vi "ReadConfigCuster.vi"(2 "error in (no error)":errorcluster, 3 "Ctrl Reference":refnum<vi>, 4 "ConfigFile (input)":T1) -> (0 "error out":errorcluster, 1 "ConfigFile (output)":T1)   [LabVIEW 2009]
uses:
  <vilib>/Utility/config.llb/Config Data RefNum.ctl
  Read Key (Double).vi
  Read Key (Boolean).vi
  Read Key (Path).vi
  Read Key (String).vi
  <vilib>/Utility/config.llb/NI_LVConfig.lvlib
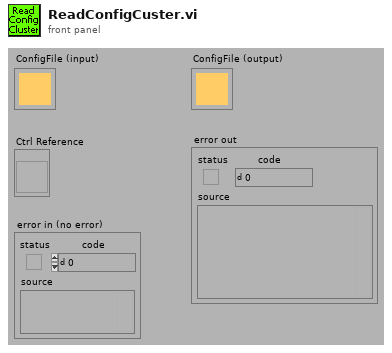
[diagram p1: front panel]
types:
  T1 = typedef "NI_LVConfig.lvlib/Config Data RefNum.ctl" = refnum<k1>
  T2 = typedef "Config Data RefNum" = refnum<k1>
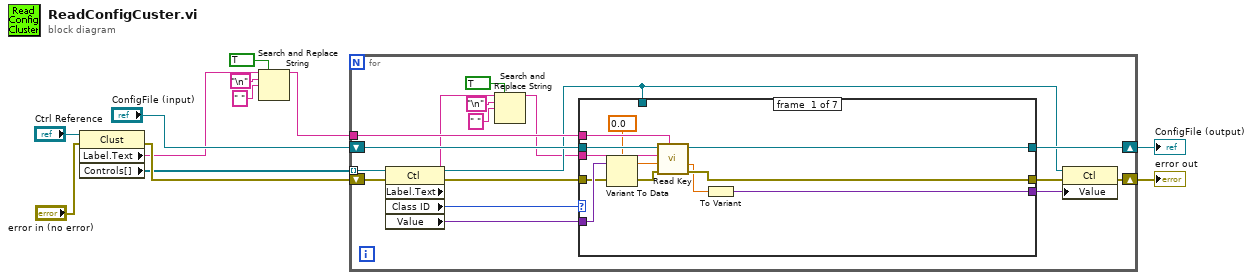
[diagram p0: block diagram]
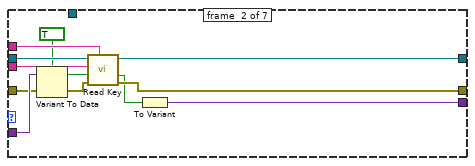
[diagram p2: hidden frame]
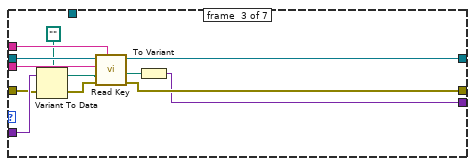
[diagram p3: hidden frame]
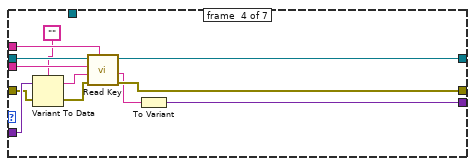
[diagram p4: hidden frame]
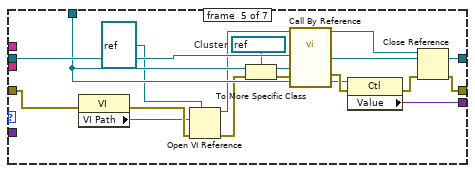
[diagram p5: hidden frame]
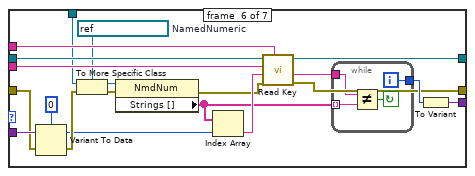
[diagram p6: hidden frame]
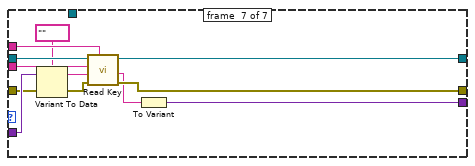
[diagram p7: hidden frame]
diagram:
  n1 = property on="Property Node" class="Clust"(reference="Ctrl Reference", error in="error in (no error)") -> (error out=w8:errorcluster, "Label.Text"=w2:string, "Controls[]"=w6:refnum<vi>[])  [unwired: 1 out]
  n2 = Search and Replace String(replace all?=TRUE ("replace all? (F)"), input string=w2, search string="\n", replace string=" ") -> (result string=w1:string)  [unwired: 4 in, 3 out]
  n3 = for {
    tunnel: w6 -> [w27] mode=indexing
    tunnel: w1 -> [w28]
    shift-right: [w23] -> w9
    shift-left: "ConfigFile (input)" -> [w24]
    shift-right: [w19] -> w12
    shift-left: w8 -> [w22]
    n4 = property on="Property Node" class="Ctl"(reference=w27, error in=w22) -> (reference out=w18:refnum<vi>, error out=w29:errorcluster, "Label.Text"=w14:string, "Class ID"=w26:u32, "Value"=w25:variant)
    n5 = Search and Replace String(replace all?=TRUE ("replace all? (F)"), input string=w14, search string="\n", replace string=" ") -> (result string=w13:string)  [unwired: 4 in, 3 out]
    n6 = case shown="27" w26 {
      tunnel: w24 -> [w41 w53 w65 w77 w94 w112 w130]
      tunnel: w29 -> [w36 w49 w61 w73 w90 w113 w126]
      tunnel: w28 -> [w40 w52 w64 w76 _ w109 w129]
      tunnel: w13 -> [w39 w51 w63 w75 _ w111 w128]
      tunnel: w25 -> [w38 w50 w62 w74 _ w114 w127]
      tunnel: [w34 w47 w59 w71 w91 w105 w124] -> w23
      tunnel: [w33 w46 w58 w70 w80 w98 w123] -> w20
      tunnel: [w31 w43 w54 w67 w89 w102 w120] -> w21
      tunnel: w18 -> [_ _ _ _ w87 w106 _]
      frame #0 {
        n7 = Variant To Data(error in=w36, Variant=w38, type=0.0) -> (error out=w35:errorcluster, data=w32:dbl)
        n8 = call-poly "Read Key.vi"("section"=w40, "error in (no error)"=w35, "default value"=w32, "key"=w39, "refnum"=w41) -> ("error out"=w33:errorcluster, "value"=w30:dbl, "refnum out"=w34:T1)  [unwired: 3 in, 1 out]
        n9 = To Variant(anything=w30) -> (Variant=w31:variant)
      }
      frame #1 {
        n10 = Variant To Data(error in=w49, Variant=w50, type=TRUE) -> (error out=w48:errorcluster, data=w44:bool)
        n11 = call-poly "Read Key.vi"("section"=w52, "error in (no error)"=w48, "default value"=w44, "key"=w51, "refnum"=w53) -> ("error out"=w46:errorcluster, "value"=w42:bool, "refnum out"=w47:T1)  [unwired: 3 in, 1 out]
        n12 = To Variant(anything=w42) -> (Variant=w43:variant)
      }
      frame #2 {
        n13 = Variant To Data(error in=w61, Variant=w62, type=path "") -> (error out=w60:errorcluster, data=w56:path)
        n14 = call-poly "Read Key.vi"("section"=w64, "error in (no error)"=w60, "default value"=w56, "key"=w63, "refnum"=w65) -> ("error out"=w58:errorcluster, "value"=w55:path, "refnum out"=w59:T1)  [unwired: 3 in, 1 out]
        n15 = To Variant(anything=w55) -> (Variant=w54:variant)
      }
      frame #3 {
        n16 = Variant To Data(error in=w73, Variant=w74, type="") -> (error out=w72:errorcluster, data=w68:string)
        n17 = call-poly "Read Key.vi"("section"=w76, "error in (no error)"=w72, "default value"=w68, "key"=w75, "refnum"=w77) -> ("error out"=w70:errorcluster, "value"=w66:string, "refnum out"=w71:T1)  [unwired: 3 in, 1 out]
        n18 = To Variant(anything=w66) -> (Variant=w67:variant)
      }
      frame #4 {
        w93 = refnum<vi> refnum  # Cluster
        n19 = property class="VI"(error in=w90) -> (error out=w86:errorcluster, "VI Path"=w85:path)  [unwired: 1 in, 1 out]
        n20 = Open VI Reference(type specifier VI Refnum (for type only)=refnum<vi> refnum, vi path=w85, error in (no error)=w86) -> (vi reference=w84:refnum<vi>, error out=w83:errorcluster)  [unwired: 3 in]
        n21 = To More Specific Class(target class=w93, reference=w87, error in=w83) -> (specific class reference=w92:refnum<vi>, error out=w79:errorcluster)
        n22 = call-by-ref "?"(reference=w84, "error in (no error)"=w79, "Ctrl Reference"=w92, "ConfigFile (input)"=w94) -> (reference out=w82:refnum<vi>, "error out"=w88:errorcluster, "ConfigFile (output)"=w91:T2)  [unwired: 1 in, 1 out]
        n23 = property on="Property Node" class="Ctl"(reference=w87, error in=w88) -> (error out=w81:errorcluster, "Value"=w89:variant)  [unwired: 1 out]
        n24 = Close Reference(reference=w82, error in (no error)=w81) -> (error out=w80:errorcluster)
      }
      frame #5 {
        w108 = refnum<vi> refnum  # NamedNumeric
        n25 = Variant To Data(error in=w113, Variant=w114, type=0) -> (error out=w101:errorcluster, data=w96:i32)
        n26 = To More Specific Class(target class=w108, reference=w106, error in=w101) -> (specific class reference=w97:refnum<vi>, error out=w107:errorcluster)
        n27 = property on="Property Node" class="NmdNum"(reference=w97, error in=w107) -> (error out=w99:errorcluster, "Strings []"=w95:string[])  [unwired: 1 out]
        n28 = Index Array(array=w95, index=w96) -> (element=w100:string)
        n29 = call-poly "Read Key.vi"("section"=w109, "error in (no error)"=w99, "default value"=w100, "key"=w111, "refnum"=w112) -> ("error out"=w98:errorcluster, "value"=w104:string, "refnum out"=w105:T1)  [unwired: 3 in, 1 out]
        n30 = while {
          tunnel: w95 -> [w117] mode=indexing
          tunnel: w104 -> [w118]
          tunnel: [w115] -> w103
          i -> [w115]
          stop <- w116 continue-if-true
          n31 = Not Equal?(x=w118, y=w117) -> (x != y?=w116:bool)
        }
        n32 = To Variant(anything=w103) -> (Variant=w102:variant)
      }
      frame #6 {
        n33 = Variant To Data(error in=w126, Variant=w127, type=tag "") -> (error out=w125:errorcluster, data=w121:tag)
        n34 = call-poly "Read Key.vi"("section"=w129, "error in (no error)"=w125, "default value"=w121, "key"=w128, "refnum"=w130) -> ("error out"=w123:errorcluster, "value"=w119:string, "refnum out"=w124:T1)  [unwired: 3 in, 1 out]
        n35 = To Variant(anything=w119) -> (Variant=w120:variant)
      }
    }
    n36 = property on="Property Node" class="Ctl"(reference=w18, error in=w20, "Value"=w21) -> (error out=w19:errorcluster)  [unwired: 1 out]
  }
  "error out" <- w12
  "ConfigFile (output)" <- w9
